vi "Animation acceleration control.vi"(0 "Visible 3 module":bool, 1 "Visible 2 module":bool, 4 "Volt 3":dbl, 6 "Volt 2":dbl, 8 "Volt 1":dbl, 10 "Acc in":dbl, 11 "Animation in":dbl) -> (3 "Acc out":dbl)   [LabVIEW 2020]
doc: "This program is used to control the animation speed - proton is moving faster with the modules voltage increasion and also only id the modules are visible. \nAcc in - provides acceleration, mostly from shift registers saved inside while loop \nVolt 1/2/3 - voltage from controls \nAcc out - the acceleration that is getting added to shift register and to position of moving proton\nVisible 2/3 module - while modules are off, speed of proton must be constant"
panel:
  # "This program is controlling protons's animation speed in dependancy of module's Voltage"
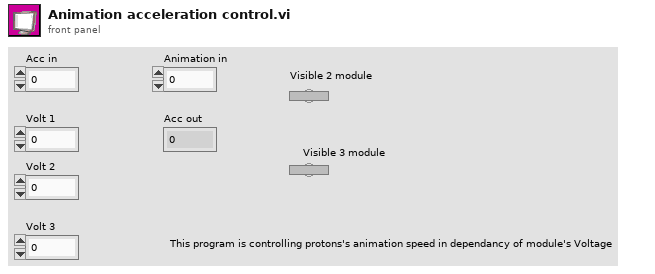
[diagram p1: front panel]
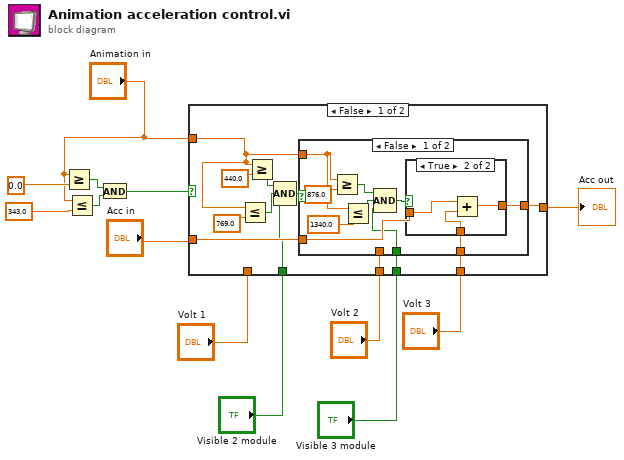
[diagram p0: block diagram]
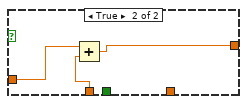
[diagram p3: hidden frame]
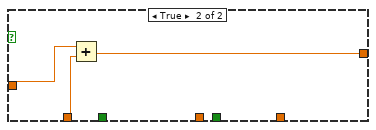
[diagram p4: hidden frame]
diagram:
  n1 = Greater Or Equal?(x="Animation in", y=0.0) -> (x >= y?=w13:bool)
  n2 = Less Or Equal?(x="Animation in", y=343.0) -> (x <= y?=w12:bool)
  n3 = And(x=w13, y=w12) -> (x .and. y?=w9:bool)
  n4 = case shown="False" w9 {
    tunnel: "Acc in" -> [w19 w45]
    tunnel: "Volt 1" -> [_ w44]
    tunnel: [w18 w43] -> w6
    tunnel: "Animation in" -> [w17 _]
    tunnel: "Volt 2" -> [w20 _]
    tunnel: "Volt 3" -> [w16 _]
    tunnel: "Visible 2 module" -> [w15 _]
    tunnel: "Visible 3 module" -> [w14 _]
    frame False {
      n5 = Less Or Equal?(x=w17, y=769.0) -> (x <= y?=w24:bool)
      n6 = Greater Or Equal?(x=w17, y=440.0) -> (x >= y?=w25:bool)
      n7 = Compound Arithmetic op=AND(w25, w24, w15) -> (w22:bool)
      n8 = case shown="False" w22 {
        tunnel: w20 -> [_ w41]
        tunnel: w19 -> [w29 w42]
        tunnel: [w28 w40] -> w18
        tunnel: w17 -> [w31 _]
        tunnel: w16 -> [w30 _]
        tunnel: w14 -> [w26 _]
        frame False {
          n9 = Greater Or Equal?(x=w31, y=876.0) -> (x >= y?=w35:bool)
          n10 = Less Or Equal?(x=w31, y=1340.0) -> (x <= y?=w34:bool)
          n11 = Compound Arithmetic op=AND(w35, w34, w26) -> (w27:bool)
          n12 = case shown="True" w27 {
            tunnel: w30 -> [_ w38]
            tunnel: w29 -> [w36 w39]
            tunnel: [w36 w37] -> w28
            frame False {
            }
            frame True {
              n13 = Add(x=w39, y=w38) -> (x+y=w37:dbl)
            }
          }
        }
        frame True {
          n14 = Add(x=w42, y=w41) -> (x+y=w40:dbl)
        }
      }
    }
    frame True {
      n15 = Add(x=w45, y=w44) -> (x+y=w43:dbl)
    }
  }
  "Acc out" <- w6
